vi "Restore Menu.vi"(8 "error in (no error)":errorcluster, 9 "Menu ref":refnum<vi>, 10 "File path":path, 11 "Monitor-Pulse in":refnum<class "Application Controller.lvclass">) -> (0 "error out":errorcluster, 1 "Section out":string, 2 "File path out":path, 3 "Monitor-Pulse out":refnum<class "Application Controller.lvclass">)   [LabVIEW 2016, in "Application Controller.lvclass"]
uses:
  Application Controller.lvclass
  C:/github/LabActor/Template Module/Template Module.lvclass
  NHMFL_Core/Libraries/Queued Listbox/Queued Listbox.xctl
  Template Module/Template Module.lvclass/Template Module.ctl
  Template Module/Read Name.vi
  <vilib>/Utility/error.llb/Error Cluster From Error Code.vi
  <vilib>/ErrorRing/Error Ring.xnode
  <vilib>/Utility/config.llb/NI_LVConfig.lvlib
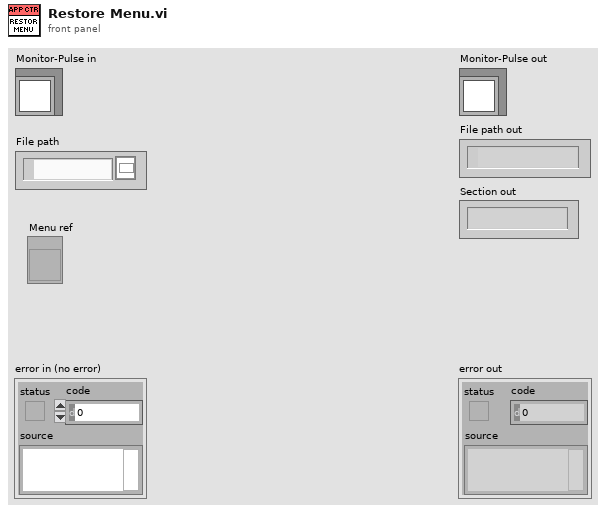
[diagram p1: front panel]
types:
  T1 = typedef "NI_LVConfig.lvlib/Config Data RefNum.ctl" = refnum<k1>
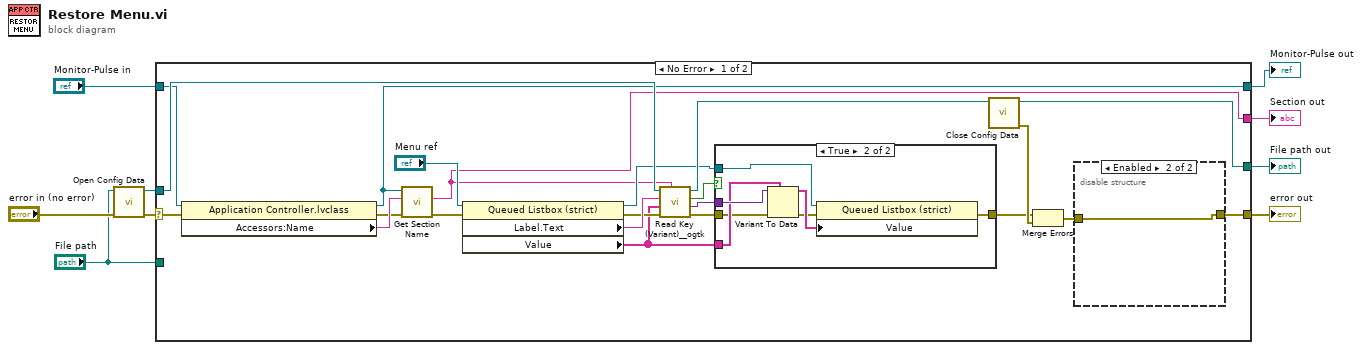
[diagram p0: block diagram]
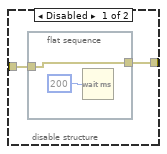
[diagram p3: hidden frame]
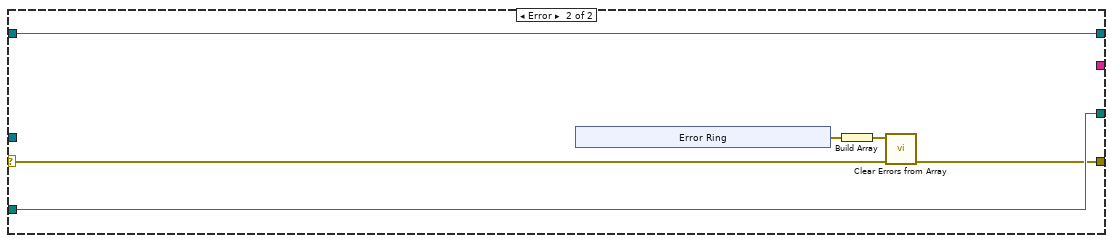
[diagram p4: hidden frame]
diagram:
  n1 = call <vilib>:"Open Config Data.vi"("error in (no error)"="error in (no error)", "configuration file path"="File path") -> ("error out"=w2:errorcluster, "refnum"=w9:T1)  [unwired: 7 in, 1 out]
  n2 = case shown="No Error" w2 {
    selector: w2 -> [w20 w46]
    tunnel: w9 -> [w31 _]
    tunnel: [w10 _] -> w8
    tunnel: [w11 w50] -> w7
    tunnel: "Monitor-Pulse in" -> [w24 w50]
    tunnel: [w12 w45] -> w5
    tunnel: [w22 w49] -> w4
    tunnel: "File path" -> [_ w49]
    frame No Error {
      n3 = property class="Application Controller.lvclass"(reference=w24, error in=w20) -> (reference out=w11:refnum<class "Application Controller.lvclass">, error out=w25:errorcluster, "Accessors:Name"=w26:string)
      n4 = call "Get Section Name.vi"("Error In"=w25, "Object name"=w26, "object"=w11) -> ("Error Out"=w21:errorcluster, "Section out"=w10:string)  [unwired: 7 in]
      n5 = property class="Queued Listbox (strict)"(reference="Menu ref", error in=w21) -> (reference out=w17:refnum<vi>, error out=w18:errorcluster, "Label.Text"=w27:string, "Value"=w15:string[])
      n6 = call <userlib>:"Read Key (Variant)__ogtk.vi"("section"=w10, "error in (no error)"=w18, "type"=w15, "key (optional)"=w27, "refnum"=w31) -> ("error out"=w14:errorcluster, "key-value"=w16:variant, "found?"=w13:bool, "refnum out"=w28:T1)  [unwired: 3 in]
      n7 = case shown="True" w13 {
        tunnel: w17 -> [_ w39]
        tunnel: w16 -> [_ w38]
        tunnel: w15 -> [_ w37]
        tunnel: w14 -> [w32 w35]
        tunnel: [w32 w33] -> w29
        frame False {
        }
        frame True {
          n8 = Variant To Data(error in=w35, type=w37, Variant=w38) -> (data=w36:string[], error out=w34:errorcluster)
          n9 = property class="Queued Listbox (strict)"(reference=w39, error in=w34, "Value"=w36) -> (error out=w33:errorcluster)  [unwired: 1 out]
        }
      }
      n10 = call <vilib>:"Close Config Data.vi"("refnum"=w28) -> ("error out"=w30:errorcluster, "file path"=w22:path)  [unwired: 9 in]
      n11 = Merge Errors(w29, w30) -> (w23:errorcluster)
      n12 = disable-structure shown="Enabled" {
        disable-tunnel: w23 -> [w41 w44]
        disable-tunnel: [w40 w44] -> w12
        frame Disabled {
          n13 = flat-sequence {
            tunnel: w41 -> [w43]
            tunnel: [w43] -> w40
            frame #0 {
              n14 = Wait (ms)(milliseconds to wait=u32 200) -> ()  [unwired: 1 out]
            }
          }
        }
        frame Enabled {
        }
      }
    }
    frame Error {
      n15 = xnode "Error Ring"() -> ("error out"=w48:errorcluster)
      n16 = Build Array(w48) -> (w47:errorcluster[])
      n17 = call "Clear Errors from Array.vi"("Error In"=w46, "Errors to clear"=w47) -> ("Error Out"=w45:errorcluster)  [unwired: 8 in, 1 out]
    }
  }
  "error out" <- w5
  "Monitor-Pulse out" <- w7
  "File path out" <- w4
  "Section out" <- w8
